vi "Compute DistanceToTarget2.vi"(6 "Robot Calibration Cluster":T1={"Camera Height on robot (in)"=34.5, "Camera Angle on the robot (deg)"=28.3, "Slope"=0.946, "Offset"=10.775} {"Offset" format="%#_13g"; "Slope" format="%#_13g"; "Camera Angle on the robot (deg)" format="%#_13g"; "Camera Height on robot (in)" format="%#_13g"}, 8 "results":T2, 10 "Field of view":dbl=120.0 format="%#_13g", 11 "Image Src":T3) -> (0 "results out":T2, 2 "Offset Angle":dbl=569.258018632146, 3 "Image Dst Out":T3)   [LabVIEW 2019]
doc: "Using the camera lens information and the real world size of the target, use trig and ratios to determine the distance to the target. Also returns the location relative to the image center in a (-1 , 1) coordinate system that may be useful for steering the robot."
uses:
  <vilib>/vision/Image Controls.llb/IMAQ Image.ctl
  Target Fields.ctl
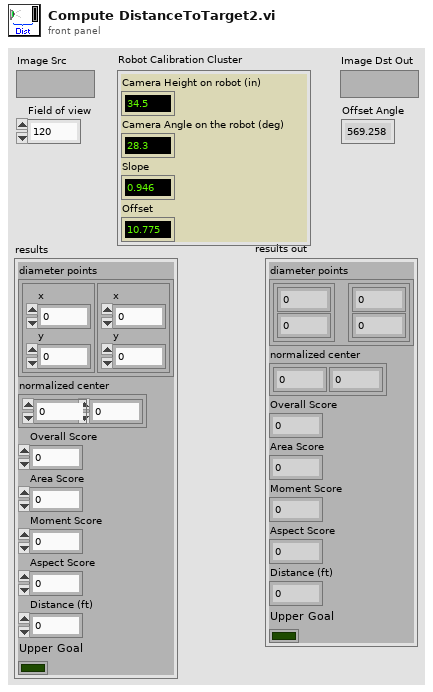
[diagram p1: front panel]
types:
  T1 = cluster{"Camera Height on robot (in)":dbl, "Camera Angle on the robot (deg)":dbl, "Slope":dbl, "Offset":dbl}
  T2 = typedef "Target Fields.ctl" = cluster{"diameter points":cluster{"first point":cluster{"x":dbl, "y":dbl}, "projected point":cluster{"x":dbl, "y":dbl}}, "normalized center":cluster{"x":dbl, "y":dbl}, "Overall Score":dbl, "Area Score":dbl, "Moment Score":dbl, "Aspect Score":dbl, "Distance (ft)":dbl, "Upper Goal":bool}
  T3 = typedef "IMAQ Image.ctl" = refnum<image>
  T4 = cluster{"first point":cluster{"x":dbl, "y":dbl}, "projected point":cluster{"x":dbl, "y":dbl}}
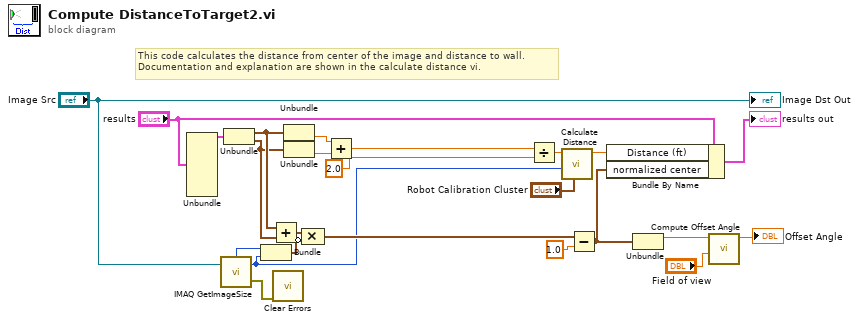
[diagram p0: block diagram]
diagram:
  # "This code calculates the distance from center of the image and distance to wall.\nDocumentation and explanation are shown in the calculate distance vi."
  n1 = Unbundle("results") -> ("diameter points"=w20:T4)  [unwired: 7 out]
  n2 = call "IMAQ GetImageSize"("Image"="Image Src") -> ("Y Resolution"=w10:i32, "X Resolution"=w11:i32, "error out"=w24:errorcluster)  [unwired: 3 in]
  n3 = Unbundle(w20) -> ("first point"=w9:cluster{"x":dbl, "y":dbl}, "projected point"=w8:cluster{"x":dbl, "y":dbl})
  n4 = Bundle("X Resolution"=w11, "Y Resolution"=w10) -> (w18:cluster{"X Resolution":i32, "Y Resolution":i32})  [unwired: 1 in]
  n5 = Add(x=w9, y=w8) -> (x+y=w17:cluster{"x":dbl, "y":dbl})
  n6 = call <vilib>:"Clear Errors.vi"("error in (no error)"=w24) -> ()  [unwired: 5 in, 2 out]
  n7 = Unbundle(w9) -> ("y"=w7:dbl)  [unwired: 1 out]
  n8 = Unbundle(w8) -> ("y"=w6:dbl)  [unwired: 1 out]
  n9 = Compound Arithmetic op=MULTIPLY(w17, invert w18) -> (w19:cluster{dbl, dbl})
  n10 = Add(x=w7, y=w6) -> (x+y=w5:dbl)
  n11 = Divide(x=w5, y=2.0) -> (x/y=w3:dbl)
  n12 = call "Calculate Distance.vi"("Robot Calibration Cluster"="Robot Calibration Cluster", "Screen resolution pixels Height (Ry)"=w10, "Middle of target from 0,0 (pixels)"=w3) -> ("Distance from target (in)"=w2:dbl)  [unwired: 8 in]
  n13 = Subtract(x=w19, y=1.0) -> (x-y=w14:cluster{dbl, dbl})
  n14 = Bundle By Name(cluster="results", "Distance (ft)"=w2, "normalized center"=w14) -> (→"results out":T2)
  n15 = Unbundle(w14) -> (w13:dbl)  [unwired: 1 out]
  n16 = call "Compute Offset Angle.vi"("Field of view"="Field of view", "Offset Normilized"=w13) -> ("Offset Angle"=→"Offset Angle":dbl)  [unwired: 9 in]
  "Image Dst Out" <- "Image Src"
